vi "ABB get path.vi"(11 "Initialize":bool) -> (3 "Path":path)   [LabVIEW 2017]
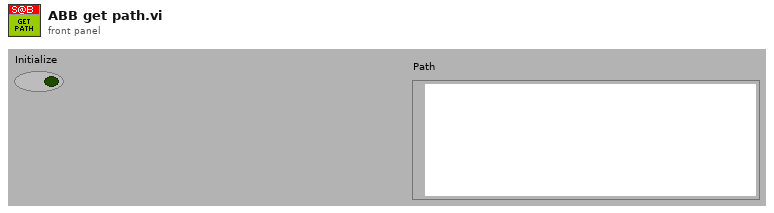
[diagram p1: front panel]
types:
  T1 = enum32{"invalid app kind", "Development System", "Run Time System", "Student Edition", "Embedded LabVIEW", "Evaluation", "Custom"}
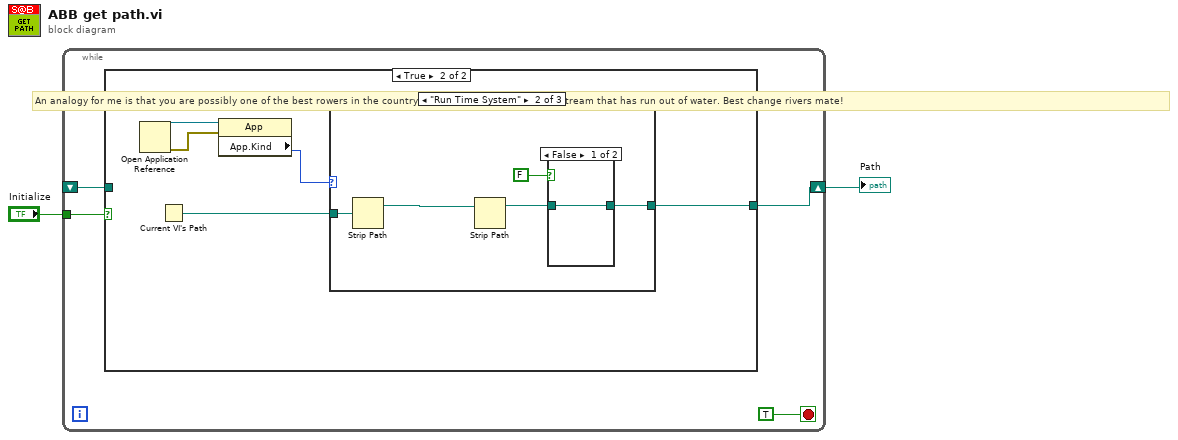
[diagram p0: block diagram]
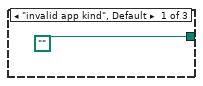
[diagram p3: hidden frame]
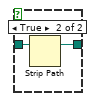
[diagram p4: hidden frame]
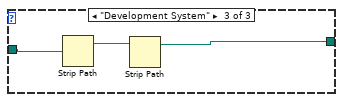
[diagram p5: hidden frame]
diagram:
  n1 = while {
    tunnel: "Initialize" -> [w5]
    shift-right: [w4] -> w1
    shift-left: _ -> [w3]
    stop <- TRUE stop-if-true
    n2 = case shown="True" w5 {
      tunnel: [w7 w8] -> w4
      tunnel: w3 -> [w7 _]
      frame False {
      }
      frame True {
        n3 = Open Application Reference() -> (0:w11:errorcluster, 3:w12:refnum<vi>)  [unwired: 4 in]
        n4 = Current VI's Path() -> (path=w9:path)
        n5 = property class="App"(reference=w12, error in=w11) -> ("App.Kind"=w10:T1)  [unwired: 2 out]
        n6 = case shown="\"Run Time System\"" w10 {
          tunnel: w9 -> [_ w18 w24]
          tunnel: [path "" w16 w22] -> w8
          frame "invalid app kind", Default {
          }
          frame "Run Time System" {
            # "An analogy for me is that you are possibly one of the best rowers in the country / world, but have rowed up a stream that has run out of water. Best change rivers mate!"
            n7 = Strip Path(path=w18) -> (stripped path=w14:path)  [unwired: 1 out]
            n8 = Strip Path(path=w14) -> (stripped path=w17:path)  [unwired: 1 out]
            n9 = case shown="False" FALSE {
              tunnel: w17 -> [w19 w21]
              tunnel: [w19 w20] -> w16
              frame False {
              }
              frame True {
                n10 = Strip Path(path=w21) -> (stripped path=w20:path)  [unwired: 1 out]
              }
            }
          }
          frame "Development System" {
            n11 = Strip Path(path=w24) -> (stripped path=w23:path)  [unwired: 1 out]
            n12 = Strip Path(path=w23) -> (stripped path=w22:path)  [unwired: 1 out]
          }
        }
      }
    }
  }
  "Path" <- w1
